vi "cRIO_EPTx_FPGA_MulInj.vi"() -> ()   [LabVIEW 2020]
uses:
  <vilib>/Powertrain Controls/Device Drivers/Engine Position Tracking/EPTx/RevA/FPGA/Controls/EPTxSimulatorConfig.ctl
  <vilib>/Powertrain Controls/Device Drivers/Engine Position Tracking/EPTx/RevA/FPGA/Controls/EPTxDebug.ctl
  <vilib>/Powertrain Controls/Device Drivers/Engine Position Tracking/EPTx/RevA/FPGA/Controls/EPTxTooth.ctl
  <vilib>/Powertrain Controls/Device Drivers/Engine Position Tracking/EPTx/RevA/FPGA/Controls/EPTxSignals.ctl
  <vilib>/Powertrain Controls/Device Drivers/Engine Position Tracking/EPTx/RevA/FPGA/Controls/EPTxSupervisor.ctl
  <vilib>/Powertrain Controls/Device Drivers/Engine Position Tracking/EPTx/RevA/FPGA/Controls/EPTxConfig.ctl
  <vilib>/Platform/TimedLoop/XDataNode/timing_clust.ctl
  <vilib>/Platform/TimedLoop/XDataNode/nitl_modes.ctl
  <vilib>/Platform/TimedLoop/XDataNode/wakeup.ctl
  <vilib>/Powertrain Controls/Device Drivers/Engine Position Tracking/EPTx/RevA/FPGA/Controls/EPTxAAPControl.ctl
  <vilib>/Powertrain Controls/Device Drivers/Engine Position Tracking/EPTx/RevA/FPGA/Controls/EPTxPatternConfig.ctl
  <vilib>/Powertrain Controls/Device Drivers/Engine Position Tracking/EPTx/RevA/FPGA/Controls/Patterns.ctl
  <vilib>/Powertrain Controls/Device Drivers/Engine Position Tracking/EPTx/RevA/FPGA/Controls/EPTxControl.ctl
  <vilib>/rvi/Emulation/niFpgaSctlEmulationGetInTimedLoop.vi
  <vilib>/rvi/Emulation/niFpgaEmulationReportErrorSimple.vi
  <vilib>/rvi/Emulation/niFpgaGetClockAttributes.vi
  <vilib>/rvi/Emulation/niFpgaCriticalErrorInLSC.vi
  <vilib>/rvi/eio/common/nirviEmuTemplateMethod_errors.vi
  <vilib>/Powertrain Controls/Device Drivers/Engine Position Tracking/EPTx/RevA/FPGA/Extras/Command Sequence - 12e.vi
  <vilib>/Platform/TimedLoop/XDataNode/XDataNode.xnode
  <vilib>/eio/EIONode/EIONode.xnode
  <vilib>/Platform/TimedLoop/XDataNode/XDNodeRunTimeDep.lvlib
  <vilib>/Powertrain Controls/Device Drivers/Engine Position Tracking/EPTx/RevA/FPGA/EPTx - RevA - FPGA.lvlib
panel:
  in  "ContinueSeq12":bool
  in  "ContinueSeq11":bool
  in  "DurationSeq12":u32
  in  "DurationSeq11":u32
  in  "CmdLevelSeq12":bool
  in  "CmdLevelSeq11":bool
  in  "ContinueSeq10":bool
  in  "ContinueSeq9":bool
  in  "CmdLevelSeq10":bool
  in  "CmdLevelSeq9":bool
  in  "DurationSeq10":u32
  in  "DurationSeq9":u32
  in  "GlobalTrigger":bool
  out "Cmd":bool
  out "Paused":bool
  out "CmdTimer":u32
  out "SeqPointer":u8
  in  "ContinueSeq8":bool
  in  "ContinueSeq7":bool
  in  "ContinueSeq6":bool
  in  "ContinueSeq5":bool
  in  "ContinueSeq4":bool
  in  "ContinueSeq3":bool
  in  "ContinueSeq2":bool
  in  "ContinueSeq1":bool
  in  "CmdLevelSeq8":bool
  in  "CmdLevelSeq7":bool
  in  "CmdLevelSeq6":bool
  in  "CmdLevelSeq5":bool
  in  "CmdLevelSeq4":bool
  in  "CmdLevelSeq3":bool
  in  "CmdLevelSeq2":bool
  in  "CmdLevelSeq1":bool
  in  "DurationSeq8":u32
  in  "DurationSeq7":u32
  in  "DurationSeq6":u32
  in  "DurationSeq5":u32
  in  "DurationSeq4":u32
  in  "DurationSeq3":u32
  in  "DurationSeq2":u32
  in  "DurationSeq1":u32
  out "OpenWinSig":bool
  in  "Delay[tick]":u32
  out "CAN_Trigger":bool
  out "Speed_Output":fxp<+/-,32,16>
  out "Cylinder_Number":u8
  in  "OpWin_Enable6":bool
  in  "OpWin_Enable5":bool
  in  "OpWin_Enable4":bool
  in  "OpWin_Enable3":bool
  in  "OpWin_Enable2":bool
  in  "OpWin_Enable1":bool
  in  "OpWin_RisingCAD6":fxp<+/-,32,16>=540.0
  in  "OpWin_FallingCAD6":fxp<+/-,32,16>=600.0
  in  "OpWin_RisingCAD5":fxp<+/-,32,16>=300.0
  in  "OpWin_FallingCAD5":fxp<+/-,32,16>=360.0
  in  "OpWin_RisingCAD4":fxp<+/-,32,16>=60.0
  in  "OpWin_FallingCAD4":fxp<+/-,32,16>=120.0
  in  "OpWin_RisingCAD3":fxp<+/-,32,16>=420.0
  in  "OpWin_FallingCAD3":fxp<+/-,32,16>=480.0
  in  "OpWin_RisingCAD2":fxp<+/-,32,16>=660.0
  in  "OpWin_FallingCAD2":fxp<+/-,32,16>=720.0
  in  "OpWin_FallingCAD1":fxp<+/-,32,16>=240.0
  in  "OpWin_RisingCAD1":fxp<+/-,32,16>=180.0
  in  "Cylinder6_H_R [CAD]":fxp<+/-,32,16>
  in  "Cylinder6_H_F [CAD]":fxp<+/-,32,16>
  in  "Cylinder5_H_R [CAD]":fxp<+/-,32,16>
  in  "Cylinder5_H_F [CAD]":fxp<+/-,32,16>
  in  "Cylinder4_H_R [CAD]":fxp<+/-,32,16>
  in  "Cylinder4_H_F [CAD]":fxp<+/-,32,16>
  in  "Cylinder3_H_R [CAD]":fxp<+/-,32,16>
  in  "Cylinder3_H_F [CAD]":fxp<+/-,32,16>
  in  "Cylinder2_H_R [CAD]":fxp<+/-,32,16>
  in  "Cylinder2_H_F [CAD]":fxp<+/-,32,16>
  in  "Cylinder1_H_F [CAD]":fxp<+/-,32,16>
  in  "Cylinder1_H_R [CAD]":fxp<+/-,32,16>
  out "Watchdog Error":bool
  in  "Aux 4":fxp<+/-,32,16>
  in  "Aux 3":fxp<+/-,32,16>
  in  "Aux 2":fxp<+/-,32,16>
  in  "Aux 1":fxp<+/-,32,16>
  in  "Aux 4 State":bool
  in  "Aux 3 State":bool
  in  "Aux 2 State":bool
  in  "Aux 1 State":bool
  in  "Sim Rate":fxp<+/-,16,7>
  in  "Watchdog":bool
  in  "Sim Enable":bool
  in  "Clear Errors":bool
  in  "Sync Enable":bool
  in  "Primary State":bool
  in  "Primary":fxp<+/-,32,16>
  in  "Address":fxp<+/-,32,16>
  out "AvgSpeed":fxp<+/-,32,16>
  out "CADRate":fxp<+/-,32,16>
  out "HistoryCAD":fxp<+/-,32,16>
  out "MaxCAD":fxp<+/-,32,16>
  out "CurrentCAD":fxp<+/-,32,16>
  out "EndCAD":fxp<+/-,32,16>
  out "StartCAD":fxp<+/-,32,16>
  out "CycleCount":fxp<+/-,64,32>
  out "Forward":bool
  out "Tooth":bool
  out "Sync 2":bool
  out "Aux Warning":bool
  out "Pattern Error":bool
  out "Ratio Error":bool
  out "Overflow":bool
  out "Stall":bool
  out "Rcvg Primary":bool
  out "Config":bool
  out "Sync":bool
  in  "EPTxConfig":T1
  out "EPTxSupervisor_FPGA":T2
  out "EPTxSignals":T3
  out "EPTxTooth":T4
  out "EPTxDebug":T5
  in  "EPTxSimulatorConfig":T6
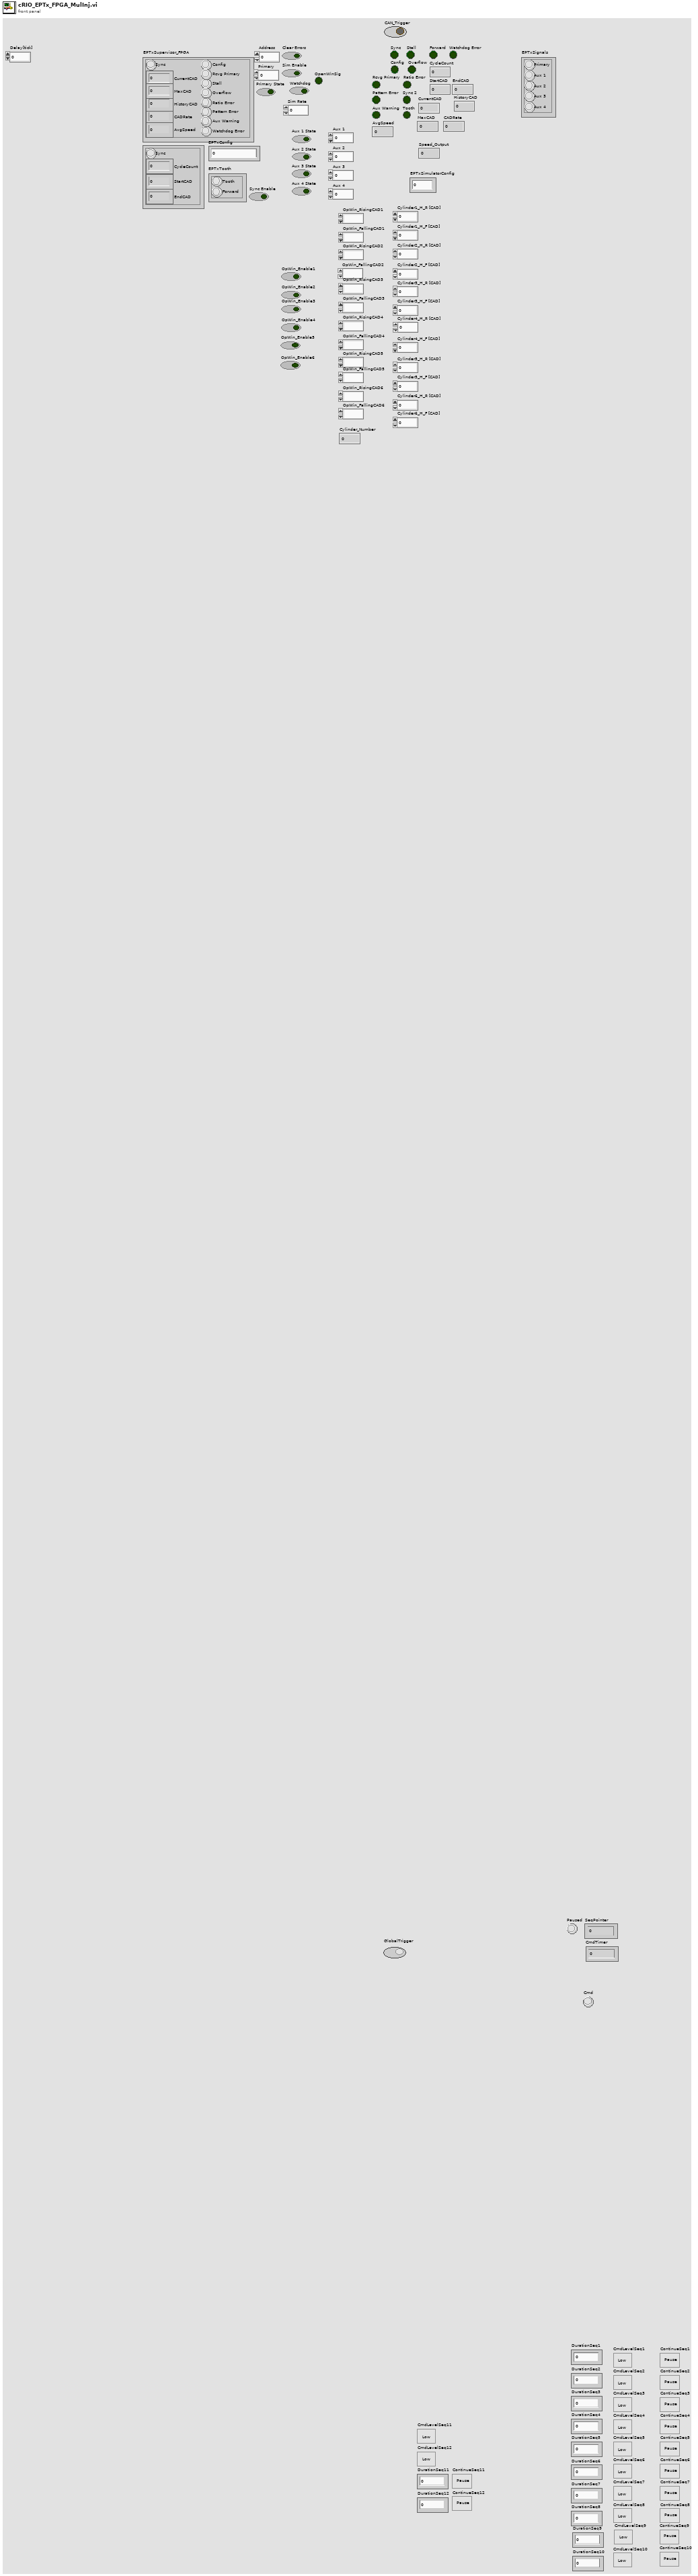
[diagram p1: front panel]
types:
  T1 = typedef "EPTx - RevA - FPGA.lvlib/EPTxConfig.ctl" = u64
  T2 = typedef "EPTx - RevA - FPGA.lvlib/EPTxSupervisor.ctl" = cluster{"Sync":bool, "CurrentCAD":fxp<+,18,11>, "MaxCAD":fxp<+,11,11>, "HistoryCAD":fxp<+,11,11>, "CADRate":fxp<+,22,8>, "AvgSpeed":fxp<+,17,15>, "Config":bool, "Rcvg Primary":bool, "Stall":bool, "Overflow":bool, "Ratio Error":bool, "Pattern Error":bool, "Aux Warning":bool, "Watchdog Error":bool}
  T3 = typedef "EPTx - RevA - FPGA.lvlib/EPTxSignals.ctl" = cluster{"Primary":bool, "Aux 1":bool, "Aux 2":bool, "Aux 3":bool, "Aux 4":bool}
  T4 = typedef "EPTx - RevA - FPGA.lvlib/EPTxTooth.ctl" = cluster{"Tooth":bool, "Forward":bool}
  T5 = typedef "EPTx - RevA - FPGA.lvlib/EPTxDebug.ctl" = cluster{"Sync":bool, "CycleCount":fxp<+,8,8>, "StartCAD":fxp<+,18,11>, "EndCAD":fxp<+,18,11>}
  T6 = typedef "EPTx - RevA - FPGA.lvlib/EPTxSimulatorConfig.ctl" = u32
  T7 = typedef "EPTx - RevA - FPGA.lvlib/EPTxAAPControl.ctl" = cluster{"Enable":bool, "RisingCAD":fxp<+,18,11>, "FallingCAD":fxp<+,18,11>}
  T8 = typedef "XDNodeRunTimeDep.lvlib/timing_clust.ctl" = cluster{"Expected End [f-1]":u64, "Actual End [f-1]":u64, "Finished Late? [f-1]":bool, "Expected End [i-1]":u64, "Actual End [i-1]":u64, "Finished Late? [i-1]":bool, "Expected Start [i]":u64, "Actual Start [i]":u64, "Expected Start [f]":u64, "Actual Start [f]":u64, "Source Name":string, "Structure Name":string, "Period":i64, "Deadline":i64, "Offset":i64, "Start":i64, "Priority":i32, "Timeout":i32, "Mode":T9, "Wakeup Reason":T10, "Error":errorcluster, "Source Type":string, "Secondary Source Type":string, "Global End Time":u64, "Global Start Time":u64, "Frame Duration":u64, "Iteration Duration":u64, "Assigned CPU":i32, "I/O Scan Engine Mode":u32}
  T9 = typedef "XDNodeRunTimeDep.lvlib/nitl_modes.ctl" = enum32{"No Change", "Process missed periods, maintain original phase", "Discard missed periods, maintain original phase", "Process missed periods, ignore original phase", "Discard missed periods, ignore original phase"}
  T10 = typedef "XDNodeRunTimeDep.lvlib/wakeup.ctl" = enum32{"Normal", "Aborted", "Asynchronous wakeup", "Timing source error", "Timed loop error", "Timeout"}
  T11 = typedef "EPTx - RevA - FPGA.lvlib/EPTxControl.ctl" = cluster{"Sync Enable":bool, "Clear Errors":bool, "Sim Enable":bool, "Sim Rate":fxp<+,24,6>, "Watchdog":bool}
  T12 = typedef "EPTx - RevA - FPGA.lvlib/Patterns.ctl" = cluster{"Primary":fxp<+,19,12>, "Primary State":bool, "Aux 1":fxp<+,19,12>, "Aux 1 State":bool, "Aux 2":fxp<+,19,12>, "Aux 2 State":bool, "Aux 3":fxp<+,19,12>, "Aux 3 State":bool, "Aux 4":fxp<+,19,12>, "Aux 4 State":bool}
  T13 = typedef "EPTx - RevA - FPGA.lvlib/EPTxPatternConfig.ctl" = cluster{"Address":fxp<+,14,14>, "Pattern":T12}
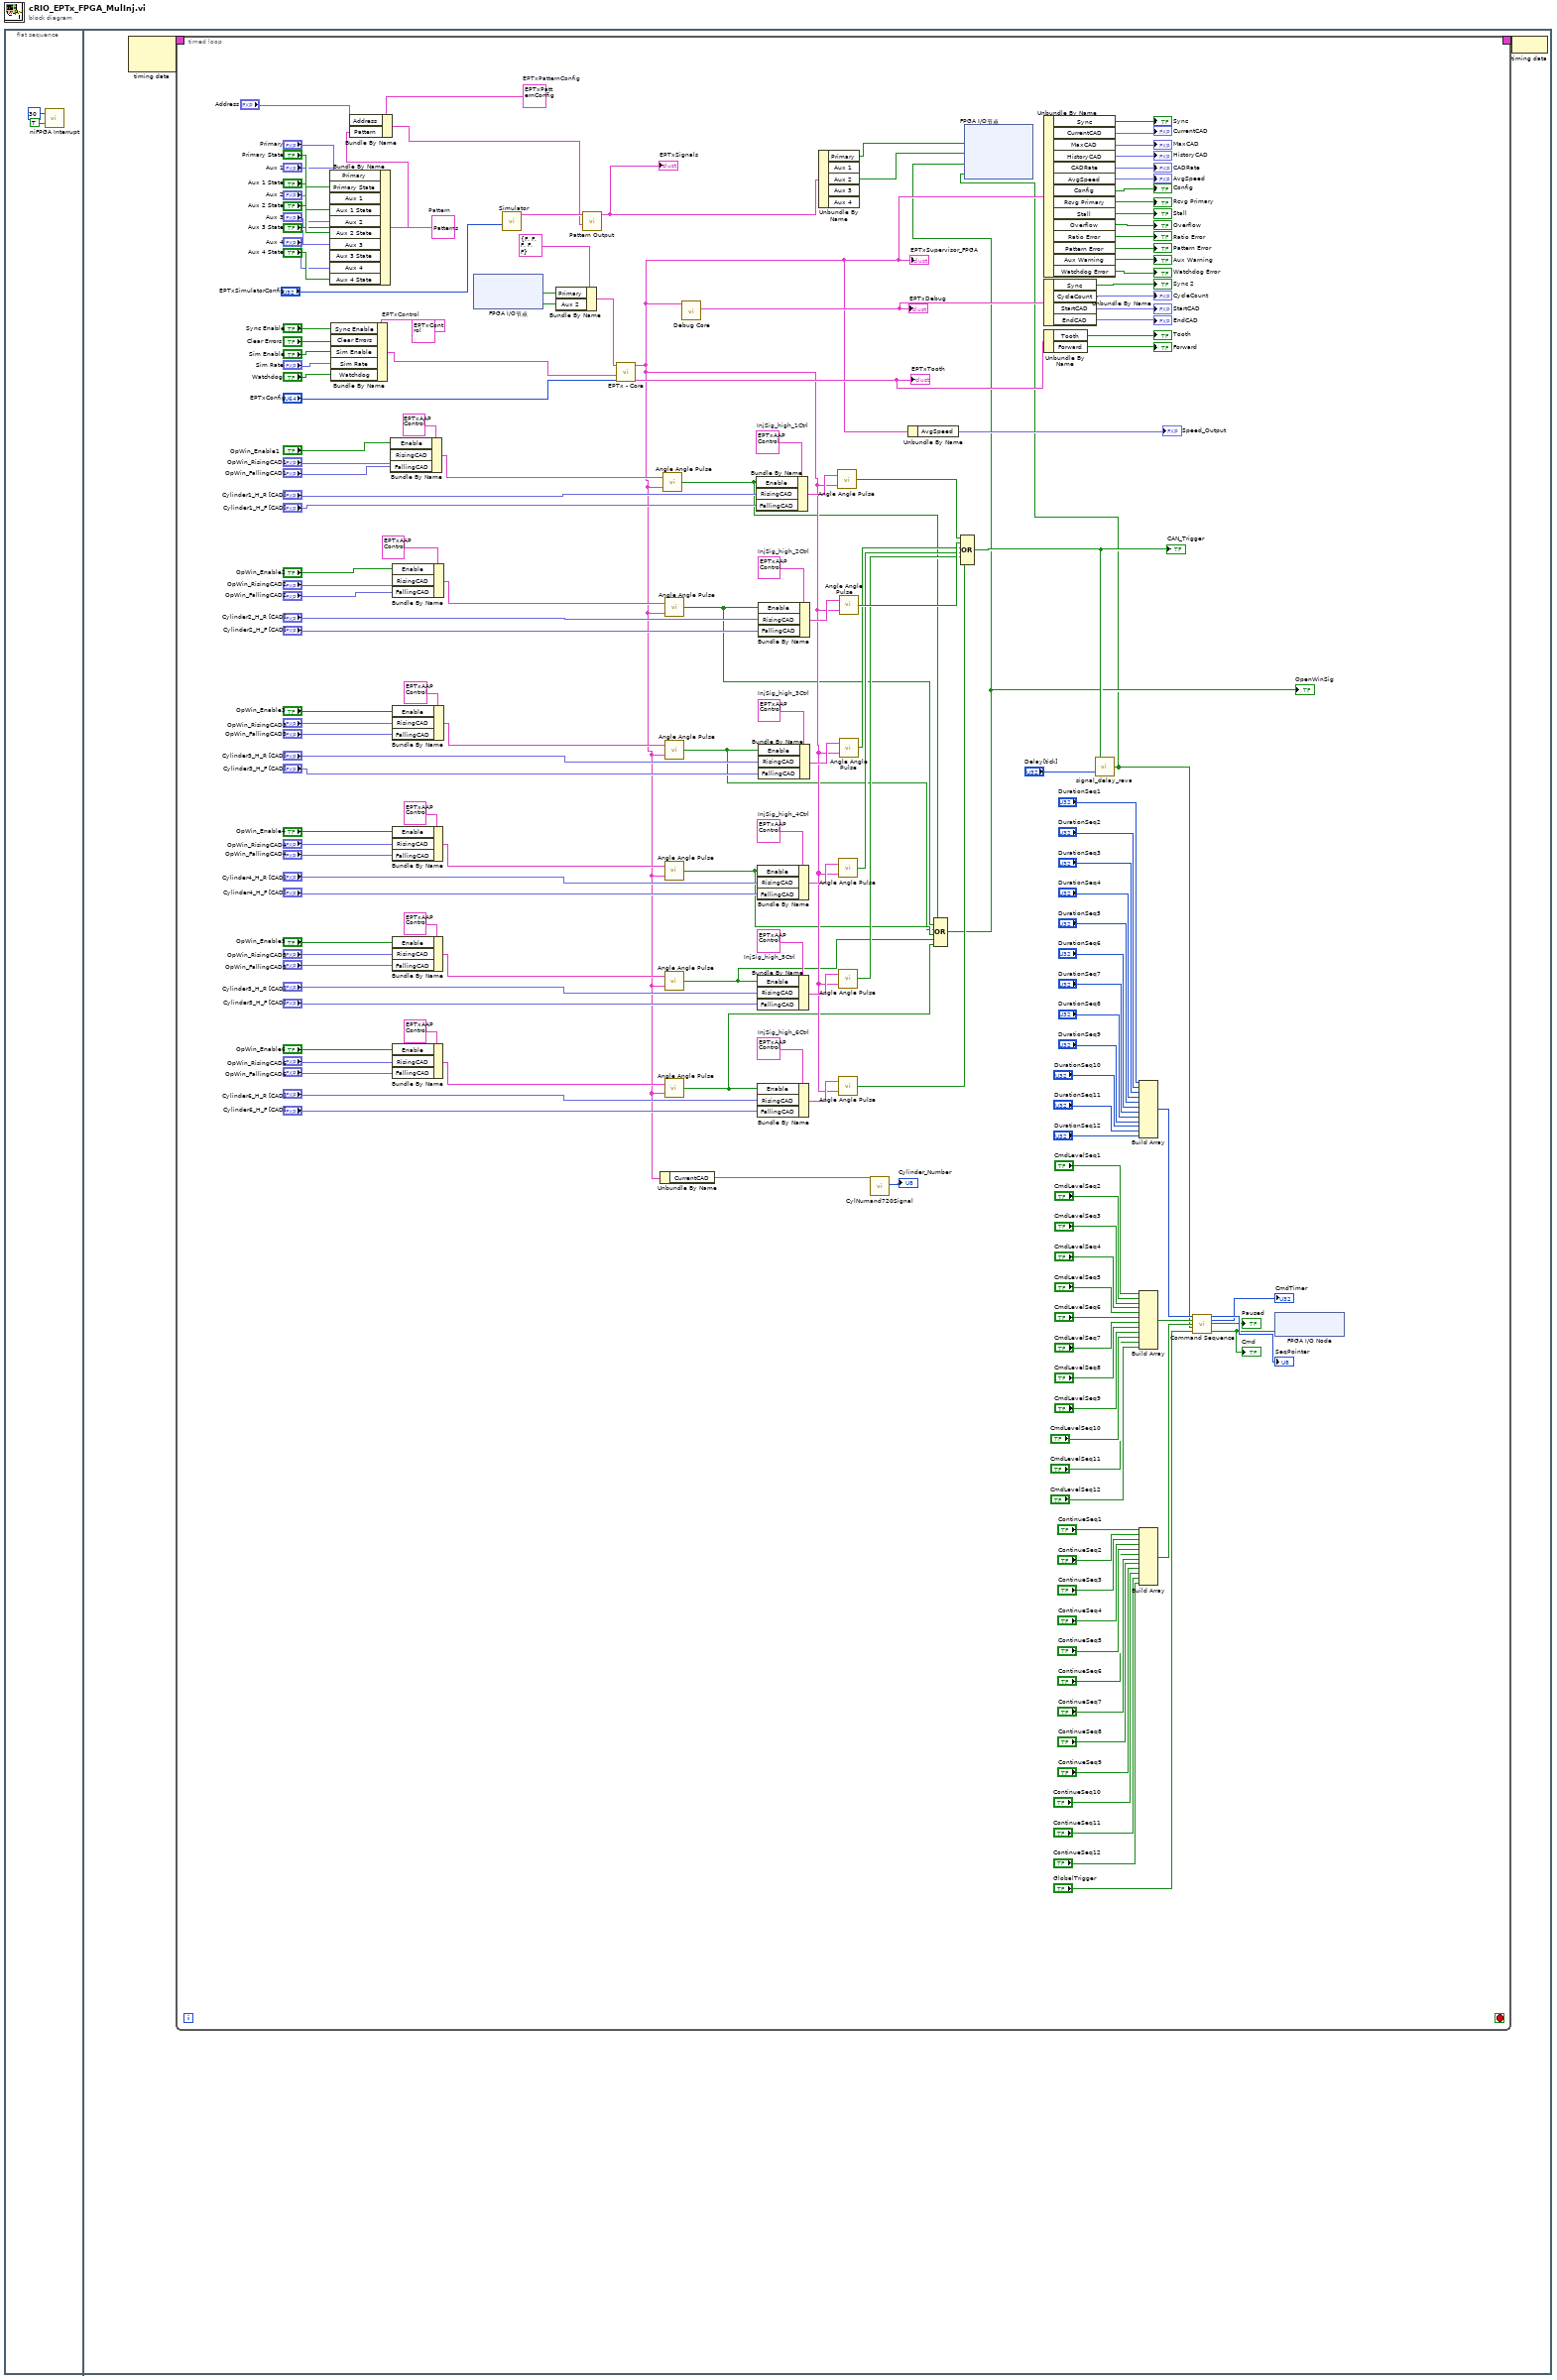
[diagram p0: block diagram]
diagram:
  n1 = flat-sequence {
    frame #0 {
      n2 = call <vilib>:"niFPGA Interrupt.vi"("Wait Until Cleared (F)"=TRUE, "IRQ Number (0)"=u8 30) -> ()  [unwired: 1 in]
    }
    frame #1 {
      n3 = node-c288() -> (w4:T8)  [unwired: 2 in]
      n4 = timed-loop {
        timing: w4 -> [_]
        timing-out: [_] -> w3
        stop <- _ stop-if-true
        w72 = T7 {"Enable"=FALSE, "RisingCAD"=0.0, "FallingCAD"=0.0}  # InjSig_high_6Ctrl
        w87 = T7 {"Enable"=FALSE, "RisingCAD"=0.0, "FallingCAD"=0.0}  # InjSig_high_5Ctrl
        w90 = T7 {"Enable"=FALSE, "RisingCAD"=0.0, "FallingCAD"=0.0}  # InjSig_high_4Ctrl
        w107 = T7 {"Enable"=FALSE, "RisingCAD"=0.0, "FallingCAD"=0.0}  # InjSig_high_3Ctrl
        w111 = T7 {"Enable"=FALSE, "RisingCAD"=0.0, "FallingCAD"=0.0}  # InjSig_high_2Ctrl
        w161 = T11 {"Sync Enable"=FALSE, "Clear Errors"=FALSE, "Sim Enable"=FALSE, "Sim Rate"=0.0, "Watchdog"=FALSE}  # EPTxControl
        w166 = T12 {"Primary"=0.0, "Primary State"=FALSE, "Aux 1"=0.0, "Aux 1 State"=FALSE, "Aux 2"=0.0, "Aux 2 State"=FALSE, "Aux 3"=0.0, "Aux 3 State"=FALSE, "Aux 4"=0.0, "Aux 4 State"=FALSE}  # Pattern
        w167 = T13 {"Address"=0.0, "Pattern"={"Primary"=0.0, "Primary State"=FALSE, "Aux 1"=0.0, "Aux 1 State"=FALSE, "Aux 2"=0.0, "Aux 2 State"=FALSE, "Aux 3"=0.0, "Aux 3 State"=FALSE, "Aux 4"=0.0, "Aux 4 State"=FALSE}}  # EPTxPatternConfig
        w170 = T7 {"Enable"=FALSE, "RisingCAD"=0.0, "FallingCAD"=0.0}  # InjSig_high_1Ctrl
        n5 = Bundle By Name(cluster=w166, "Primary"="Primary", "Primary State"="Primary State", "Aux 1"="Aux 1", "Aux 1 State"="Aux 1 State", "Aux 2"="Aux 2", "Aux 2 State"="Aux 2 State", "Aux 3"="Aux 3", "Aux 3 State"="Aux 3 State", "Aux 4"="Aux 4", "Aux 4 State"="Aux 4 State") -> (w165:T12)
        n6 = Bundle By Name(cluster=w161, "Sync Enable"="Sync Enable", "Clear Errors"="Clear Errors", "Sim Enable"="Sim Enable", "Sim Rate"="Sim Rate", "Watchdog"="Watchdog") -> (w160:T11)
        n7 = Bundle By Name(cluster=w167, "Address"="Address", "Pattern"=w165) -> (w164:T13)
        n8 = Bundle By Name(cluster=T7 {"Enable"=FALSE, "RisingCAD"=0.0, "FallingCAD"=0.0} ("AAPControl_1str"), "Enable"="OpWin_Enable1", "RisingCAD"="OpWin_RisingCAD1", "FallingCAD"="OpWin_FallingCAD1") -> (w162:T7)
        n9 = Bundle By Name(cluster=T7 {"Enable"=FALSE, "RisingCAD"=0.0, "FallingCAD"=0.0} ("AAPControl_1str"), "Enable"="OpWin_Enable4", "RisingCAD"="OpWin_RisingCAD4", "FallingCAD"="OpWin_FallingCAD4") -> (w92:T7)
        n10 = Bundle By Name(cluster=T7 {"Enable"=FALSE, "RisingCAD"=0.0, "FallingCAD"=0.0} ("AAPControl_1str"), "Enable"="OpWin_Enable5", "RisingCAD"="OpWin_RisingCAD5", "FallingCAD"="OpWin_FallingCAD5") -> (w85:T7)
        n11 = Bundle By Name(cluster=T7 {"Enable"=FALSE, "RisingCAD"=0.0, "FallingCAD"=0.0} ("AAPControl_1str"), "Enable"="OpWin_Enable6", "RisingCAD"="OpWin_RisingCAD6", "FallingCAD"="OpWin_FallingCAD6") -> (w74:T7)
        n12 = Bundle By Name(cluster=T7 {"Enable"=FALSE, "RisingCAD"=0.0, "FallingCAD"=0.0} ("AAPControl_1str"), "Enable"="OpWin_Enable2", "RisingCAD"="OpWin_RisingCAD2", "FallingCAD"="OpWin_FallingCAD2") -> (w113:T7)
        n13 = Bundle By Name(cluster=T7 {"Enable"=FALSE, "RisingCAD"=0.0, "FallingCAD"=0.0} ("AAPControl_1str"), "Enable"="OpWin_Enable3", "RisingCAD"="OpWin_RisingCAD3", "FallingCAD"="OpWin_FallingCAD3") -> (w105:T7)
        n14 = xnode "FPGA I/O节点"() -> ("Mod7/DIO0"=w60:bool, "Mod7/DIO1"=w59:bool)  [unwired: 2 in, 2 out]
        n15 = call <vilib>:"Simulator.vi"("EPTxSimulatorConfig"="EPTxSimulatorConfig") -> ("EPTxSupervisor"=w175:T2)  [unwired: 10 in]
        n16 = Bundle By Name(cluster=T3 {"Primary"=FALSE, "Aux 1"=FALSE, "Aux 2"=FALSE, "Aux 3"=FALSE, "Aux 4"=FALSE} ("EPTxSignals"), "Primary"=w60, "Aux 2"=w59) -> (w61:T3)
        n17 = call <vilib>:"Pattern Output.vi"("EPTxPatternConfig"=w164, "EPTxSupervisor"=w175) -> ("PatternOutput"=w173:T3)  [unwired: 9 in]
        "EPTxSignals" <- w173
        n18 = call <vilib>:"EPTx - Core.vi"("EPTxConfig"="EPTxConfig", "EPTxControl"=w160, "EPTxSignals"=w61) -> ("EPTxTooth"=w168:T4, "EPTxSupervisor"=w65:T2)  [unwired: 7 in]
        "EPTxSupervisor_FPGA" <- w65
        "EPTxTooth" <- w168
        n19 = Unbundle By Name(w65) -> ("CurrentCAD"=w66:fxp<+,18,11>)
        n20 = call <vilib>:"Angle Angle Pulse.vi"("EPTxSupervisor"=w65, "AAPControl"=w162) -> ("AAP"=w51:bool)
        n21 = call <vilib>:"Angle Angle Pulse.vi"("EPTxSupervisor"=w65, "AAPControl"=w92) -> ("AAP"=w54:bool)
        n22 = call <vilib>:"Angle Angle Pulse.vi"("EPTxSupervisor"=w65, "AAPControl"=w85) -> ("AAP"=w55:bool)
        n23 = call <vilib>:"Angle Angle Pulse.vi"("EPTxSupervisor"=w65, "AAPControl"=w74) -> ("AAP"=w56:bool)
        n24 = call <vilib>:"Angle Angle Pulse.vi"("EPTxSupervisor"=w65, "AAPControl"=w113) -> ("AAP"=w52:bool)
        n25 = call <vilib>:"Angle Angle Pulse.vi"("EPTxSupervisor"=w65, "AAPControl"=w105) -> ("AAP"=w53:bool)
        n26 = call <vilib>:"Debug Core.vi"("EPTxSupervisor"=w65) -> ("EPTxDebug"=w169:T5)  [unwired: 10 in]
        "EPTxDebug" <- w169
        n27 = Bundle By Name(cluster=w170, "Enable"=w51, "RisingCAD"="Cylinder1_H_R [CAD]", "FallingCAD"="Cylinder1_H_F [CAD]") -> (w171:T7)
        n28 = Bundle By Name(cluster=w90, "Enable"=w54, "RisingCAD"="Cylinder4_H_R [CAD]", "FallingCAD"="Cylinder4_H_F [CAD]") -> (w89:T7)
        n29 = Bundle By Name(cluster=w87, "Enable"=w55, "RisingCAD"="Cylinder5_H_R [CAD]", "FallingCAD"="Cylinder5_H_F [CAD]") -> (w88:T7)
        n30 = Bundle By Name(cluster=w72, "Enable"=w56, "RisingCAD"="Cylinder6_H_R [CAD]", "FallingCAD"="Cylinder6_H_F [CAD]") -> (w71:T7)
        n31 = Bundle By Name(cluster=w111, "Enable"=w52, "RisingCAD"="Cylinder2_H_R [CAD]", "FallingCAD"="Cylinder2_H_F [CAD]") -> (w110:T7)
        n32 = Bundle By Name(cluster=w107, "Enable"=w53, "RisingCAD"="Cylinder3_H_R [CAD]", "FallingCAD"="Cylinder3_H_F [CAD]") -> (w108:T7)
        n33 = Unbundle By Name(w173) -> ("Primary"=w172:bool, "Aux 2"=w63:bool)  [unwired: 3 out]
        n34 = call <vilib>:"Angle Angle Pulse.vi"("EPTxSupervisor"=w65, "AAPControl"=w171) -> ("AAP"=w109:bool)
        n35 = call <vilib>:"Angle Angle Pulse.vi"("EPTxSupervisor"=w65, "AAPControl"=w89) -> ("AAP"=w70:bool)
        n36 = call <vilib>:"Angle Angle Pulse.vi"("EPTxSupervisor"=w65, "AAPControl"=w88) -> ("AAP"=w69:bool)
        n37 = call <vilib>:"Angle Angle Pulse.vi"("EPTxSupervisor"=w65, "AAPControl"=w71) -> ("AAP"=w68:bool)
        n38 = call <vilib>:"Angle Angle Pulse.vi"("EPTxSupervisor"=w65, "AAPControl"=w110) -> ("AAP"=w99:bool)
        n39 = call <vilib>:"Angle Angle Pulse.vi"("EPTxSupervisor"=w65, "AAPControl"=w108) -> ("AAP"=w98:bool)
        n40 = call "CylNumand720Signal.vi"("CurrentCAD"=w66) -> ("数值输入控件"=→"Cylinder_Number":u8)  [unwired: 10 in]
        n41 = Unbundle By Name(w65) -> ("AvgSpeed"=→"Speed_Output":fxp<+,17,15>)
        n42 = Compound Arithmetic op=OR ("复合运算")(w51, w52, w53, w54, w55, w56) -> (w50:bool)
        "OpenWinSig" <- w50
        n43 = Compound Arithmetic op=OR ("复合运算")(w109, w99, w98, w70, w69, w68) -> (w58:bool)
        "CAN_Trigger" <- w58
        n44 = Unbundle By Name(w169) -> ("Sync"=→"Sync 2":bool, "CycleCount"=→"CycleCount":fxp<+,8,8>, "StartCAD"=→"StartCAD":fxp<+,18,11>, "EndCAD"=→"EndCAD":fxp<+,18,11>)
        n45 = Unbundle By Name(w65) -> ("Sync"=→"Sync":bool, "CurrentCAD"=→"CurrentCAD":fxp<+,18,11>, "MaxCAD"=→"MaxCAD":fxp<+,11,11>, "HistoryCAD"=→"HistoryCAD":fxp<+,11,11>, "CADRate"=→"CADRate":fxp<+,22,8>, "AvgSpeed"=→"AvgSpeed":fxp<+,17,15>, "Config"=→"Config":bool, "Rcvg Primary"=→"Rcvg Primary":bool, "Stall"=→"Stall":bool, "Overflow"=→"Overflow":bool, "Ratio Error"=→"Ratio Error":bool, "Pattern Error"=→"Pattern Error":bool, "Aux Warning"=→"Aux Warning":bool, "Watchdog Error"=→"Watchdog Error":bool)
        n46 = Unbundle By Name(w168) -> ("Tooth"=→"Tooth":bool, "Forward"=→"Forward":bool)
        n47 = call <vilib>:"signal_delay_reva.vi"("Delay"="Delay[tick]", "InpSig"=w58) -> ("OutSig"=w17:bool)
        n48 = xnode "FPGA I/O节点"("Mod6/DIO0"=w172, "Mod6/DIO1"=w63, "Mod6/DIO2"=w50, "Mod6/DIO5"=w17) -> ()  [unwired: 4 in, 4 out]
        n49 = Build Array("DurationSeq1", "DurationSeq2", "DurationSeq3", "DurationSeq4", "DurationSeq5", "DurationSeq6", "DurationSeq7", "DurationSeq8", "DurationSeq9", "DurationSeq10", "DurationSeq11", "DurationSeq12") -> (w41:u32[])
        n50 = Build Array("CmdLevelSeq1", "CmdLevelSeq2", "CmdLevelSeq3", "CmdLevelSeq4", "CmdLevelSeq5", "CmdLevelSeq6", "CmdLevelSeq7", "CmdLevelSeq8", "CmdLevelSeq9", "CmdLevelSeq10", "CmdLevelSeq11", "CmdLevelSeq12") -> (w24:bool[])
        n51 = Build Array("ContinueSeq1", "ContinueSeq2", "ContinueSeq3", "ContinueSeq4", "ContinueSeq5", "ContinueSeq6", "ContinueSeq7", "ContinueSeq8", "ContinueSeq9", "ContinueSeq10", "ContinueSeq11", "ContinueSeq12") -> (w23:bool[])
        n52 = call-poly <vilib>:"Command Sequence.vi"("DurationSeq"=w41, "CmdLevelSeq"=w24, "ContinueSeq"=w23, "SeqReset"=w17, "GlobalTrigger"="GlobalTrigger") -> ("SeqPointer"=→"SeqPointer":u8, "CmdTimer"=→"CmdTimer":u32, "Paused"=→"Paused":bool, "Cmd"=w18:bool)  [unwired: 7 in]
        "Cmd" <- w18
        n53 = xnode "FPGA I/O Node"("Mod6/DIO3"=w18) -> ()  [unwired: 1 in, 1 out]
      }
      n54 = node-c288(w3) -> ()
    }
  }
